vi "Histogram Min & Max Percentiles.vi"(8 "error in (no error)":errorcluster, 9 "Min":dbl, 10 "Max":dbl, 11 "Histogram":cluster{"X":dbl[], "Y":dbl[]}) -> (0 "error out":errorcluster, 1 "Percentile below Min":dbl, 2 "Percentile above Max":dbl)   [LabVIEW 2021, in "Histograms.lvlib"]
uses:
  Histograms.lvlib
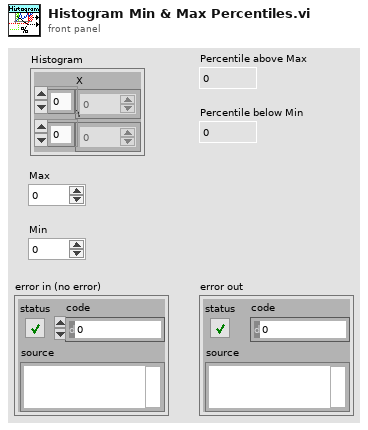
[diagram p1: front panel]
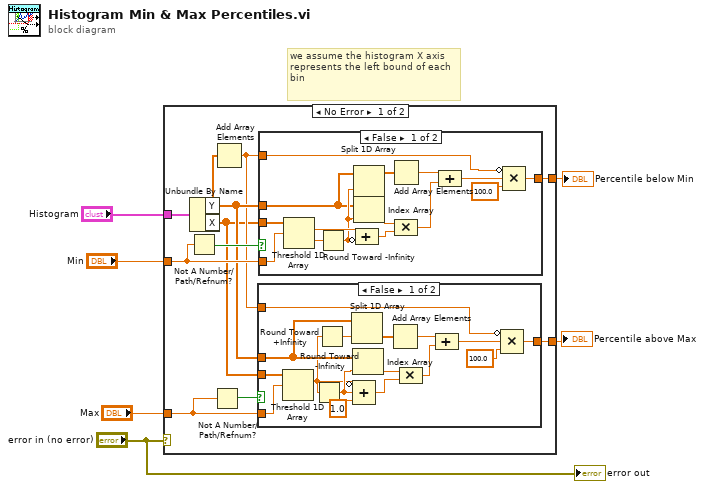
[diagram p0: block diagram]
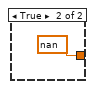
[diagram p2: hidden frame]
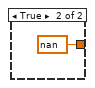
[diagram p3: hidden frame]
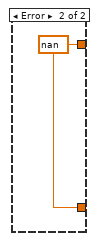
[diagram p4: hidden frame]
diagram:
  # "we assume the histogram X axis represents the left bound of each bin"
  n1 = case shown="No Error" "error in (no error)" {
    tunnel: "Histogram" -> [w16 _]
    tunnel: "Min" -> [w15 _]
    tunnel: [w13 w49] -> w4
    tunnel: "Max" -> [w11 _]
    tunnel: [w7 w49] -> w2
    frame No Error {
      n2 = Not A Number/Path/Refnum?(number/path/refnum=w15) -> (NaN/Path/Refnum?=w14:bool)
      n3 = Unbundle By Name(w16) -> ("Y"=w10:dbl[], "X"=w8:dbl[])
      n4 = Not A Number/Path/Refnum?(number/path/refnum=w11) -> (NaN/Path/Refnum?=w12:bool)
      n5 = Add Array Elements(numeric array=w10) -> (sum=w9:dbl)
      n6 = case shown="False" w12 {
        tunnel: w8 -> [w32 _]
        tunnel: w11 -> [w31 _]
        tunnel: w10 -> [w27 _]
        tunnel: w9 -> [w23 _]
        tunnel: [w21 nan] -> w7
        frame False {
          n7 = Threshold 1D Array(2:w31, 3:w32) -> (0:w19:dbl)  [unwired: 1 in]
          n8 = Round Toward -Infinity(1:w19) -> (0:w28:dbl)
          n9 = Round Toward +Infinity(x=w19) -> (ceil(x): smallest int >= x=w18:dbl)
          n10 = Split 1D Array(array=w27, index=w18) -> (second subarray=w17:dbl[])  [unwired: 1 out]
          n11 = Index Array(array=w27, index=w28) -> (element=w30:dbl)
          n12 = Compound Arithmetic op=ADD(invert w19, w28, 1.0 ("value")) -> (w29:dbl)
          n13 = Add Array Elements(numeric array=w17) -> (sum=w26:dbl)
          n14 = Compound Arithmetic op=MULTIPLY(w30, w29) -> (w25:dbl)
          n15 = Compound Arithmetic op=ADD(w26, w25) -> (w24:dbl)
          n16 = Compound Arithmetic op=MULTIPLY(invert w23, w24, 100.0 ("value")) -> (w21:dbl)
        }
        frame True {
        }
      }
      n17 = case shown="False" w14 {
        tunnel: w8 -> [w47 _]
        tunnel: w15 -> [w46 _]
        tunnel: w10 -> [w41 _]
        tunnel: w9 -> [w36 _]
        tunnel: [w34 nan] -> w13
        frame False {
          n18 = Threshold 1D Array(2:w46, 3:w47) -> (0:w45:dbl)  [unwired: 1 in]
          n19 = Round Toward -Infinity(1:w45) -> (0:w42:dbl)
          n20 = Split 1D Array(array=w41, index=w42) -> (first subarray=w40:dbl[])  [unwired: 1 out]
          n21 = Index Array(array=w41, index=w42) -> (element=w44:dbl)
          n22 = Compound Arithmetic op=ADD(w45, invert w42) -> (w43:dbl)
          n23 = Add Array Elements(numeric array=w40) -> (sum=w39:dbl)
          n24 = Compound Arithmetic op=MULTIPLY(w44, w43) -> (w38:dbl)
          n25 = Compound Arithmetic op=ADD(w39, w38) -> (w37:dbl)
          n26 = Compound Arithmetic op=MULTIPLY(invert w36, w37, 100.0 ("value")) -> (w34:dbl)
        }
        frame True {
        }
      }
    }
    frame Error {
      w49 = nan
    }
  }
  "Percentile below Min" <- w4
  "Percentile above Max" <- w2
  "error out" <- "error in (no error)"
